vi "Procedure Parameters Example (A).vi"() -> ()   [LabVIEW 2011]
uses:
  C:/Program Files/Metrohm Autolab/Autolab SDK 1.10/EcoChemie.Autolab.Sdk.dll
  EcoChemie.Autolab.Sdk.dll
panel:
  out "error out":errorcluster
  out "DoubleGet":dbl
  out "IntGet":i32
  in  "DoubleSet":dbl
  in  "IntSet":i32
  in  "SetBool":bool
  in  "SetDouble":bool
  in  "SetInt":bool
  in  "Command Parameter":string(combo)
  in  "Command":string(combo)
  in  "EnumSet":i32(ring) items=["Off", "On"]
  in  "SetEnum":bool
  out "EnumGet":i32(ring) items=["Off", "On"]
  in  "Value 2":bool
  out "0, 1":i16
  in  "Stop":bool
  in  "Procedure":path=path "Standard Nova Procedures/Cyclic voltammetry.nox"
  in  "Load":bool
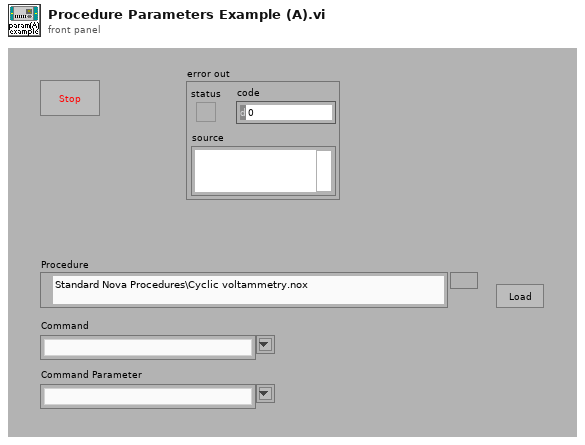
[diagram p1: front panel]
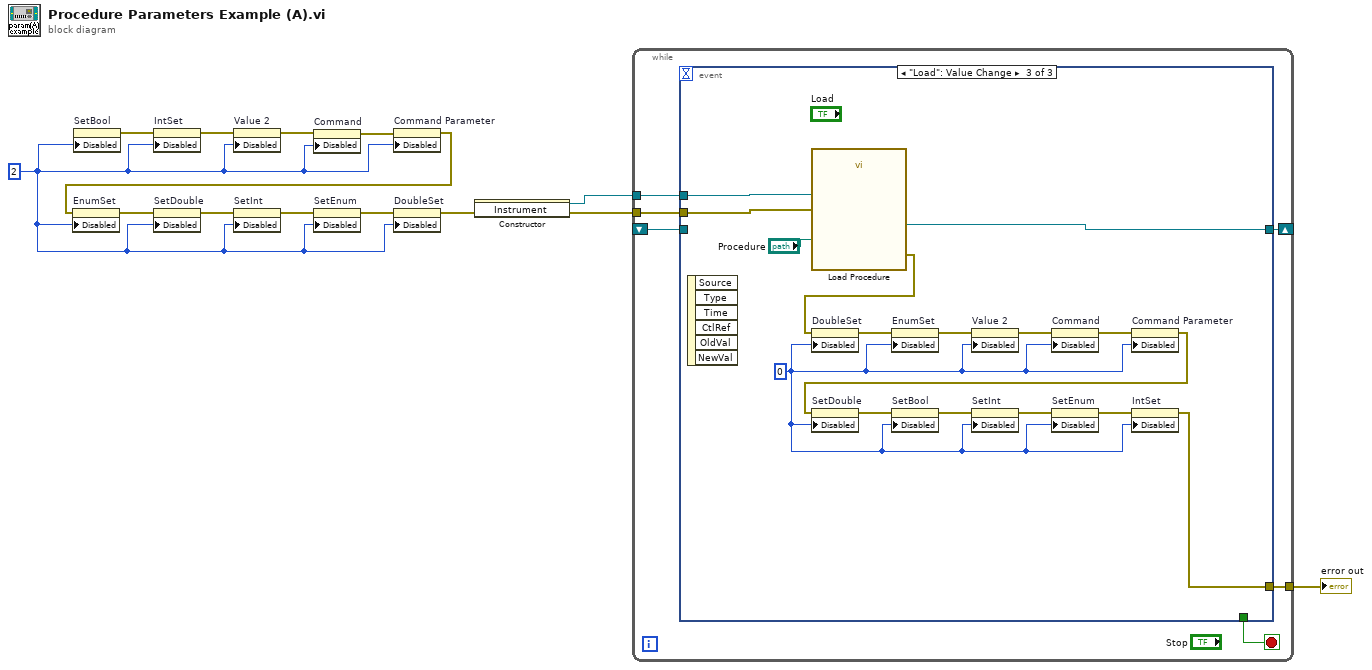
[diagram p0: block diagram]
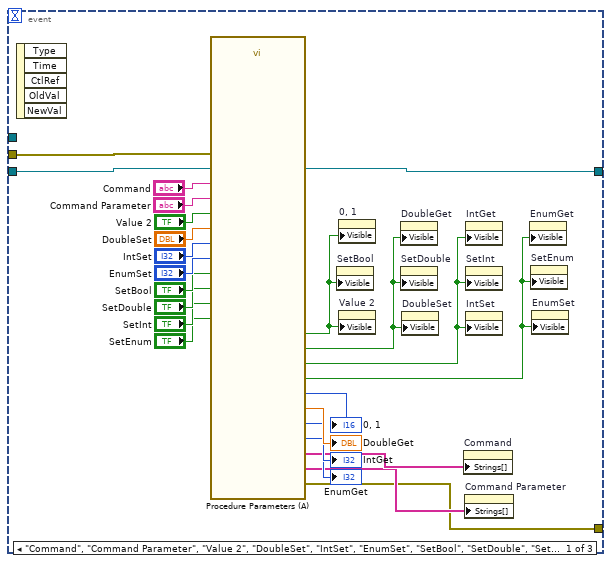
[diagram p2: hidden frame]
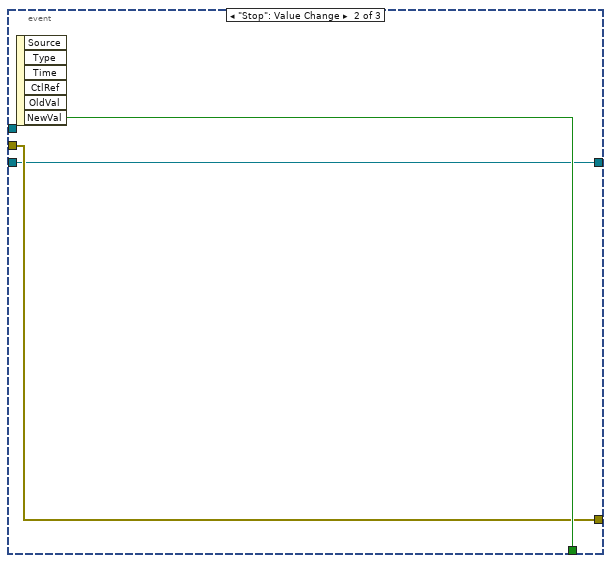
[diagram p3: hidden frame]
diagram:
  w14 = u8 2 ("Disabled")
  n1 = property on="SetBool" class="Bool (strict)"("Disabled"=w14) -> (error out=w13:errorcluster)  [unwired: 2 in, 1 out]
  n2 = property on="IntSet" class="DigNum (strict)"(error in=w13, "Disabled"=w14) -> (error out=w12:errorcluster)  [unwired: 1 in, 1 out]
  n3 = property on="Value 2" class="Bool (strict)"(error in=w12, "Disabled"=w14) -> (error out=w11:errorcluster)  [unwired: 1 in, 1 out]
  n4 = property on="Command" class="CmbBox"(error in=w11, "Disabled"=w14) -> (error out=w10:errorcluster)  [unwired: 1 in, 1 out]
  n5 = property on="Command Parameter" class="CmbBox"(error in=w10, "Disabled"=w14) -> (error out=w9:errorcluster)  [unwired: 1 in, 1 out]
  n6 = property on="EnumSet" class="Ring (strict)"(error in=w9, "Disabled"=w14) -> (error out=w8:errorcluster)  [unwired: 1 in, 1 out]
  n7 = property on="SetDouble" class="Bool (strict)"(error in=w8, "Disabled"=w14) -> (error out=w7:errorcluster)  [unwired: 1 in, 1 out]
  n8 = property on="SetInt" class="Bool (strict)"(error in=w7, "Disabled"=w14) -> (error out=w6:errorcluster)  [unwired: 1 in, 1 out]
  n9 = property on="SetEnum" class="Bool (strict)"(error in=w6, "Disabled"=w14) -> (error out=w5:errorcluster)  [unwired: 1 in, 1 out]
  n10 = property on="DoubleSet" class="DigNum (strict)"(error in=w5, "Disabled"=w14) -> (error out=w2:errorcluster)  [unwired: 1 in, 1 out]
  n11 = constructor class="Instrument"(error in=w2) -> (reference out=w3:refnum<k24>, error out=w1:errorcluster)  [unwired: 2 in, 1 out]
  n12 = while {
    tunnel: w1 -> [w20]
    tunnel: [w19] -> w4
    shift-right: [w17] -> _
    shift-left: _ -> [w16]
    tunnel: w3 -> [w15]
    stop <- w18 stop-if-true
    n13 = event shown="[2] \"Load\": Value Change" {
      selector: _ -> [_ _ _]
      dyn-events: _ -> [_ _ _]
      timeout: _ -> [_ _ _]
      tunnel: w20 -> [w43 w45 w60]
      tunnel: [w26 w45 w49] -> w19
      tunnel: [_ w46 _] -> w18
      tunnel: [w21 w44 w61] -> w17
      tunnel: w16 -> [w21 w44 _]
      tunnel: w15 -> [_ _ w59]
      event "Command", "Command Parameter", "Value 2", "DoubleSet", "IntSet", "EnumSet", "SetBool", "SetDouble", "SetInt", "SetEnum": Value Change {
        n14 = event-data() -> ()  [unwired: 1 in, 5 out]
        n15 = call "Procedure Parameters (A).vi"("LoadProcedure"=w21, "Command"="Command", "Command Parameter"="Command Parameter", "EnumSet"="EnumSet", "DoubleSet"="DoubleSet", "IntSet"="IntSet", "BoolSet"="Value 2", "SetEnum"="SetEnum", "SetDouble"="SetDouble", "SetInt"="SetInt", "SetBool"="SetBool", "error in (no error)"=w43) -> ("error out"=w26:errorcluster, "IntGet"=→"IntGet":i32, "0, 1"=→"0, 1":i16, "EnumGet"=→"EnumGet":i32, "DoubleGet"=→"DoubleGet":dbl, "Command Names"=w28:string[], "Command Parameters"=w27:string[], "VisibleEnum"=w22:bool, "VisibleInt"=w23:bool, "VisibleDouble"=w24:bool, "VisableBool"=w25:bool)  [unwired: 5 in]
        n16 = property on="SetBool" class="Bool (strict)"("Visible"=w25) -> ()  [unwired: 2 in, 2 out]
        n17 = property on="0, 1" class="DigNum (strict)"("Visible"=w25) -> ()  [unwired: 2 in, 2 out]
        n18 = property on="Value 2" class="Bool (strict)"("Visible"=w25) -> ()  [unwired: 2 in, 2 out]
        n19 = property on="DoubleGet" class="DigNum (strict)"("Visible"=w24) -> ()  [unwired: 2 in, 2 out]
        n20 = property on="SetDouble" class="Bool (strict)"("Visible"=w24) -> ()  [unwired: 2 in, 2 out]
        n21 = property on="DoubleSet" class="DigNum (strict)"("Visible"=w24) -> ()  [unwired: 2 in, 2 out]
        n22 = property on="Command" class="CmbBox"("Strings[]"=w28) -> ()  [unwired: 2 in, 2 out]
        n23 = property on="Command Parameter" class="CmbBox"("Strings[]"=w27) -> ()  [unwired: 2 in, 2 out]
        n24 = property on="IntGet" class="DigNum (strict)"("Visible"=w23) -> ()  [unwired: 2 in, 2 out]
        n25 = property on="SetInt" class="Bool (strict)"("Visible"=w23) -> ()  [unwired: 2 in, 2 out]
        n26 = property on="IntSet" class="DigNum (strict)"("Visible"=w23) -> ()  [unwired: 2 in, 2 out]
        n27 = property on="EnumGet" class="Ring (strict)"("Visible"=w22) -> ()  [unwired: 2 in, 2 out]
        n28 = property on="SetEnum" class="Bool (strict)"("Visible"=w22) -> ()  [unwired: 2 in, 2 out]
        n29 = property on="EnumSet" class="Ring (strict)"("Visible"=w22) -> ()  [unwired: 2 in, 2 out]
      }
      event "Stop": Value Change {
        n30 = event-data() -> ("NewVal"=w46:bool)  [unwired: 1 in, 5 out]
      }
      event "Load": Value Change {
        w48 = u8 0 ("Disabled")
        n31 = event-data() -> ()  [unwired: 1 in, 6 out]
        n32 = call "Load Procedure.vi"("error in (no error)"=w60, "Procedure"="Procedure", "Instrument"=w59) -> ("error out"=w47:errorcluster, "LoadProcedure"=w61:refnum<k24>)  [unwired: 5 in, 2 out]
        n33 = property on="DoubleSet" class="DigNum (strict)"(error in=w47, "Disabled"=w48) -> (error out=w58:errorcluster)  [unwired: 1 in, 1 out]
        n34 = property on="EnumSet" class="Ring (strict)"(error in=w58, "Disabled"=w48) -> (error out=w57:errorcluster)  [unwired: 1 in, 1 out]
        n35 = property on="Value 2" class="Bool (strict)"(error in=w57, "Disabled"=w48) -> (error out=w56:errorcluster)  [unwired: 1 in, 1 out]
        n36 = property on="Command" class="CmbBox"(error in=w56, "Disabled"=w48) -> (error out=w55:errorcluster)  [unwired: 1 in, 1 out]
        n37 = property on="Command Parameter" class="CmbBox"(error in=w55, "Disabled"=w48) -> (error out=w54:errorcluster)  [unwired: 1 in, 1 out]
        n38 = property on="SetDouble" class="Bool (strict)"(error in=w54, "Disabled"=w48) -> (error out=w53:errorcluster)  [unwired: 1 in, 1 out]
        n39 = property on="SetBool" class="Bool (strict)"(error in=w53, "Disabled"=w48) -> (error out=w52:errorcluster)  [unwired: 1 in, 1 out]
        n40 = property on="SetInt" class="Bool (strict)"(error in=w52, "Disabled"=w48) -> (error out=w51:errorcluster)  [unwired: 1 in, 1 out]
        n41 = property on="SetEnum" class="Bool (strict)"(error in=w51, "Disabled"=w48) -> (error out=w50:errorcluster)  [unwired: 1 in, 1 out]
        n42 = property on="IntSet" class="DigNum (strict)"(error in=w50, "Disabled"=w48) -> (error out=w49:errorcluster)  [unwired: 1 in, 1 out]
      }
    }
  }
  "error out" <- w4
